vi "Close Calling VI's Windows.vi"(4 "error in":errorcluster, 6 "level (1)":i32=1, 7 "close (T)":bool) -> (0 "error out":errorcluster)   [LabVIEW 2009, in "Tools_String.lvlib"]
uses:
  Tools_String.lvlib
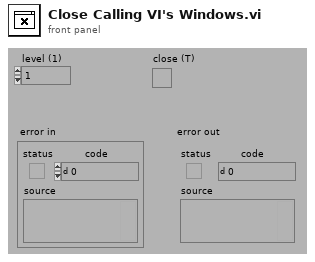
[diagram p1: front panel]
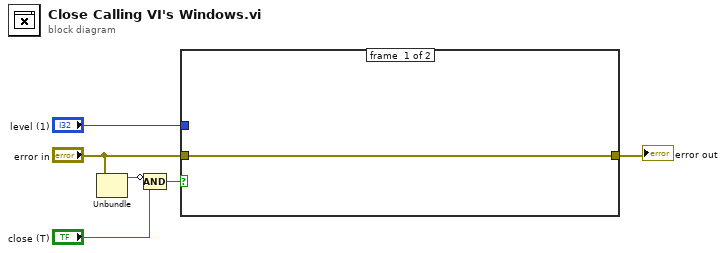
[diagram p0: block diagram]
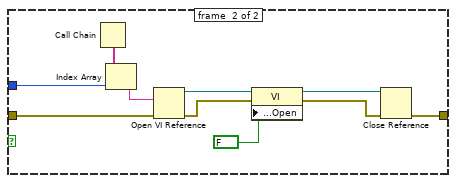
[diagram p2: hidden frame]
diagram:
  n1 = Unbundle("error in") -> ("status"=w6:bool)  [unwired: 2 out]
  n2 = Compound Arithmetic op=AND(invert w6, "close (T)") -> (w3:bool)
  n3 = case shown="True" w3 {
    tunnel: "error in" -> [w7 w10]
    tunnel: [w7 w9] -> w2
    tunnel: "level (1)" -> [_ w8]
    frame #0 {
    }
    frame #1 {
      n4 = Call Chain() -> (call chain=w17:string[])
      n5 = Index Array(array=w17, index=w8) -> (element=w11:string)
      n6 = Open VI Reference(vi path=w11, error in (no error)=w10) -> (vi reference=w16:refnum<vi>, error out=w13:errorcluster)  [unwired: 4 out]
      n7 = property class="VI"(reference=w16, error in=w13, "Front Panel Window:Open"=FALSE ("Front Panel.Open")) -> (reference out=w14:refnum<vi>, error out=w12:errorcluster)
      n8 = Close Reference(reference=w14, error in (no error)=w12) -> (error out=w9:errorcluster)
    }
  }
  "error out" <- w2
